vi "Read Ch Select.vi"(8 "error in (no error)":errorcluster, 11 "Temp Control in":refnum<class "Temp Control.lvclass">) -> (0 "error out":errorcluster, 2 "Ch Select":i32[](array[numeric]), 3 "Temp Control out":refnum<class "Temp Control.lvclass">)   [LabVIEW 2022 SP3, in "Temp Control.lvclass"]
uses:
  Temp Control.lvclass
  Temp Control.lvclass/Temp Control.ctl
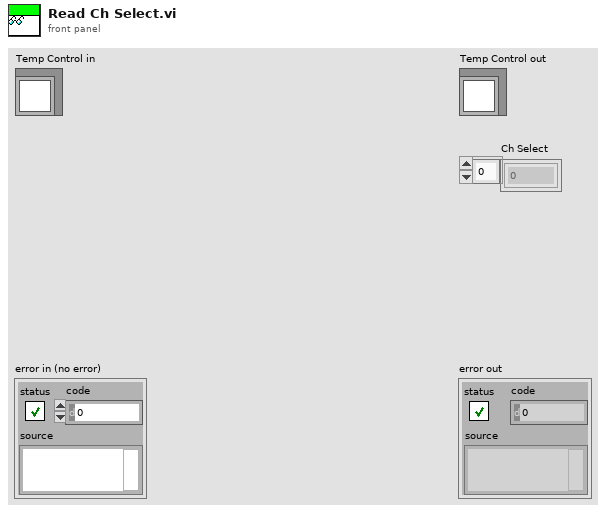
[diagram p1: front panel]
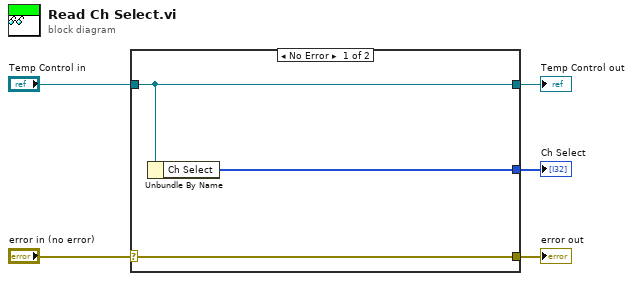
[diagram p0: block diagram]
diagram:
  n1 = case shown="No Error" "error in (no error)" {
    selector: "error in (no error)" -> [w8 w9]
    tunnel: [w8 w9] -> w4
    tunnel: [w7 w10] -> w2
    tunnel: "Temp Control in" -> [w7 w10]
    tunnel: [w6 _] -> w1
    frame No Error {
      n2 = Unbundle By Name(w7) -> ("Ch Select"=w6:i32[])
    }
    frame Error {
    }
  }
  "error out" <- w4
  "Temp Control out" <- w2
  "Ch Select" <- w1
